vi "Get Plugin Directory Path.vi"() -> (3 "Plugin Directory":path)   [LabVIEW 2020, in "Utilities.lvlib"]
uses:
  Utilities.lvlib
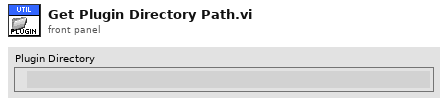
[diagram p1: front panel]
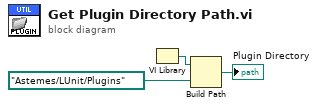
[diagram p0: block diagram]
diagram:
  n1 = VI Library() -> (path=w3:path)
  n2 = Build Path(base path=w3, name or relative path=path "Astemes/LUnit/Plugins") -> (appended path=→"Plugin Directory":path)
